vi "PhotonPNPResult_pack_OLD.vi"(11 "PNP_Result":T1={"IsPresent"=FALSE, "bestReprojErr"=0.0, "altReprojErr"=0.0, "ambiguity"=0.0, "Best"={"TRANSLATION3D"={"X"=0.0, "Y"=0.0, "Z"=0.0}, "ROTATION3D"={"Q_quaternion"={"R"=1.0, "V"=[0.0, 0.0, 0.0]}}, "XF"=FALSE}, "Alt"={"TRANSLATION3D"={"X"=0.0, "Y"=0.0, "Z"=0.0}, "ROTATION3D"={"Q_quaternion"={"R"=1.0, "V"=[0.0, 0.0, 0.0]}}, "XF"=FALSE}} {"Alt"."TRANSLATION3D"."Z" format="%14.3f"; "Alt"."TRANSLATION3D"."Y" format="%14.3f"; "Alt"."TRANSLATION3D"."X" format="%14.3f"; "Best"."TRANSLATION3D"."Z" format="%14.3f"; "Best"."TRANSLATION3D"."Y" format="%14.3f"; "Best"."TRANSLATION3D"."X" format="%14.3f"}) -> (3 "RawData Out":u8[](array[numeric]))   [LabVIEW 2019, in "PhotonVisionLib.lvlib"]
doc: "Encode a PNP Result cluster into an array of bytes.\n\nInputs:\n - PNP_Result -- PNP_Result cluster.\n\nOutputs:\n - RawDataOut -- Byte array containing the encoded data."
uses:
  TypeDef/PhotonPNPResultType.ctl
  <vilib>/Rock Robotics/WPI/ThirdParty/JAS_Junk/TrajLib/TypeDef/TRANSFORM3D.ctl
  <vilib>/Rock Robotics/WPI/ThirdParty/JAS_Junk/TrajLib/TypeDef/TRANSLATION3D.ctl
  <vilib>/Rock Robotics/WPI/ThirdParty/JAS_Junk/TrajLib/TypeDef/ROTATION3D.ctl
  <vilib>/Rock Robotics/WPI/ThirdParty/JAS_Junk/TrajLib/TypeDef/QUATERNION.ctl
  <vilib>/Rock Robotics/WPI/ThirdParty/JAS_Junk/TrajLib/VI/Transform3d_GetXYZ.vi
  <vilib>/Rock Robotics/WPI/ThirdParty/JAS_Junk/TrajLib/VI/Transform3d_GetRotation3d.vi
  <vilib>/Rock Robotics/WPI/ThirdParty/JAS_Junk/TrajLib/VI/Rotation3d_GetQuaterion.vi
  <vilib>/Rock Robotics/WPI/ThirdParty/JAS_Junk/TrajLib/VI/Quaternion_Get_All.vi
  <vilib>/Rock Robotics/WPI/ThirdParty/JAS_Junk/TrajLib/VI/Transform3d_GetTranslation3d.vi
  <vilib>/Rock Robotics/WPI/ThirdParty/JAS_Junk/TrajLib/VI/Translation3d_GetXYZ.vi
  PhotonVisionLib.lvlib
  <vilib>/Rock Robotics/WPI/ThirdParty/JAS_Junk/TrajLib/Trajectory_Library.lvlib
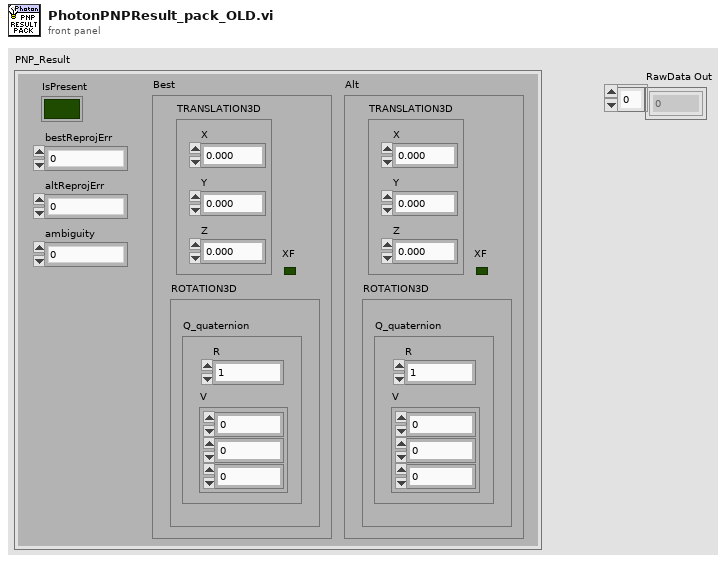
[diagram p1: front panel]
types:
  T1 = typedef "PhotonVisionLib.lvlib/PhotonPNPResultType.ctl" = cluster{"IsPresent":bool, "bestReprojErr":dbl, "altReprojErr":dbl, "ambiguity":dbl, "Best":T2, "Alt":T2}
  T2 = typedef "Trajectory_Library.lvlib/TRANSFORM3D.ctl" = cluster{"TRANSLATION3D":T3, "ROTATION3D":T4, "XF":bool}
  T3 = typedef "Trajectory_Library.lvlib/TRANSLATION3D.ctl" = cluster{"X":dbl, "Y":dbl, "Z":dbl}
  T4 = typedef "Trajectory_Library.lvlib/ROTATION3D.ctl" = cluster{"Q_quaternion":T5}
  T5 = typedef "Trajectory_Library.lvlib/QUATERNION.ctl" = cluster{"R":dbl, "V":dbl[]}
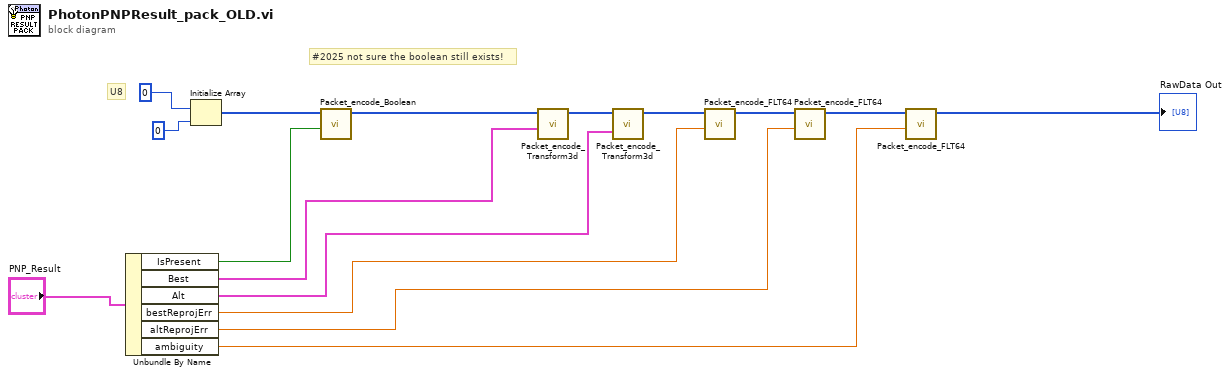
[diagram p0: block diagram]
diagram:
  # "#2025 not sure the boolean still exists!"
  # "U8"
  n1 = Unbundle By Name("PNP_Result") -> ("IsPresent"=w11:bool, "Best"=w9:T2, "Alt"=w8:T2, "bestReprojErr"=w7:dbl, "altReprojErr"=w6:dbl, "ambiguity"=w5:dbl)
  n2 = Initialize Array(u8 0 ("element"), 0 ("dimension size")) -> (w13:u8[])
  n3 = call "Packet_encode_Boolean.vi"("Boolean_Value"=w11, "RawData In"=w13) -> ("RawData Out"=w12:u8[])  [unwired: 9 in]
  n4 = call "Packet_encode_Transform3d.vi"("Transform3d Value"=w9, "RawData In"=w12) -> ("RawData Out"=w4:u8[])  [unwired: 9 in]
  n5 = call "Packet_encode_Transform3d.vi"("Transform3d Value"=w8, "RawData In"=w4) -> ("RawData Out"=w3:u8[])  [unwired: 9 in]
  n6 = call "Packet_encode_FLT64.vi"("FLT64_Value"=w7, "RawData In"=w3) -> ("RawData Out"=w2:u8[])  [unwired: 9 in]
  n7 = call "Packet_encode_FLT64.vi"("FLT64_Value"=w6, "RawData In"=w2) -> ("RawData Out"=w1:u8[])  [unwired: 9 in]
  n8 = call "Packet_encode_FLT64.vi"("FLT64_Value"=w5, "RawData In"=w1) -> ("RawData Out"=→"RawData Out":u8[])  [unwired: 9 in]
